vi "StopMotion.vi"(8 "error in (no error)":errorcluster, 9 "Axis, 1 - 4":i32=1, 11 "UI MotionStatus in":refnum<class "UI MotionStatus.lvclass">) -> (0 "error out":errorcluster, 3 "UI MotionStatus out":refnum<class "UI MotionStatus.lvclass">)   [LabVIEW 2018, in "UI MotionStatus.lvclass"]
uses:
  UI MotionStatus.lvclass
  UI MotionStatus.lvclass/UI MotionStatus.ctl
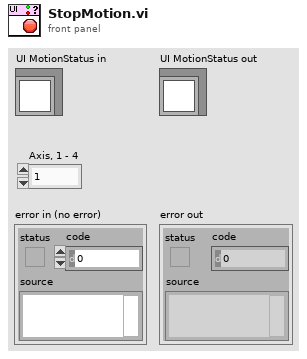
[diagram p1: front panel]
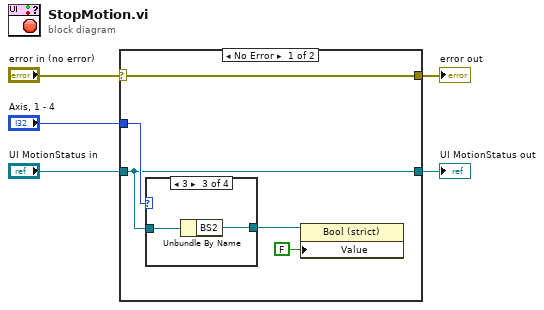
[diagram p0: block diagram]
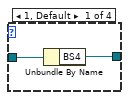
[diagram p2: hidden frame]
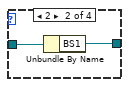
[diagram p3: hidden frame]
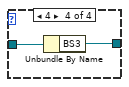
[diagram p4: hidden frame]
diagram:
  n1 = case shown="No Error" "error in (no error)" {
    selector: "error in (no error)" -> [w10 w20]
    tunnel: [w10 w20] -> w4
    tunnel: [w8 w19] -> w2
    tunnel: "UI MotionStatus in" -> [w8 w19]
    tunnel: "Axis, 1 - 4" -> [w9 _]
    frame No Error {
      n2 = case shown="3" w9 {
        tunnel: w8 -> [w12 w14 w16 w18]
        tunnel: [w11 w13 w15 w17] -> w7
        frame 1, Default {
          n3 = Unbundle By Name(w12) -> ("BS4"=w11:refnum<vi>)
        }
        frame 2 {
          n4 = Unbundle By Name(w14) -> ("BS1"=w13:refnum<vi>)
        }
        frame 3 {
          n5 = Unbundle By Name(w16) -> ("BS2"=w15:refnum<vi>)
        }
        frame 4 {
          n6 = Unbundle By Name(w18) -> ("BS3"=w17:refnum<vi>)
        }
      }
      n7 = property class="Bool (strict)"(reference=w7, "Value"=FALSE) -> ()  [unwired: 1 in, 2 out]
    }
    frame Error {
    }
  }
  "error out" <- w4
  "UI MotionStatus out" <- w2
